vi "Write Log_folder path.vi"(8 "error in (no error)":errorcluster, 10 "Log_folder path":path, 11 "Log in":refnum<class "Log.lvclass">) -> (0 "error out":errorcluster, 3 "Log out":refnum<class "Log.lvclass">)   [LabVIEW 2024, in "Log.lvclass"]
uses:
  Log.lvclass
  Log.lvclass/Log.ctl
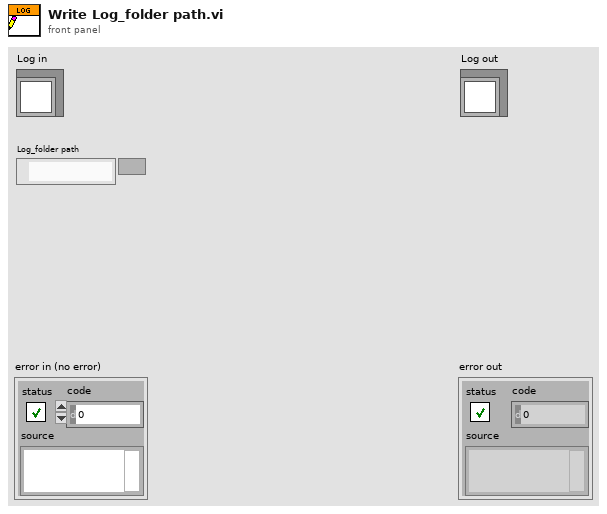
[diagram p1: front panel]
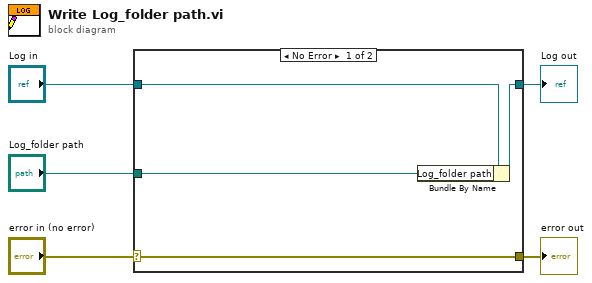
[diagram p0: block diagram]
diagram:
  n1 = case shown="No Error" "error in (no error)" {
    selector: "error in (no error)" -> [w9 w10]
    tunnel: [w9 w10] -> w4
    tunnel: [w7 w11] -> w2
    tunnel: "Log in" -> [w8 w11]
    tunnel: "Log_folder path" -> [w6 _]
    frame No Error {
      n2 = Bundle By Name(cluster=w8, "Log_folder path"=w6) -> (w7:refnum<class "Log.lvclass">)
    }
    frame Error {
    }
  }
  "error out" <- w4
  "Log out" <- w2
